vi "Load Temp.vi"(8 "error in (no error)":errorcluster, 10 "temp file name":string="ic_sparc.cfg", 11 "Channel in":refnum<class "Channel.lvclass">) -> (0 "error out":errorcluster, 3 "Channel out":refnum<class "Channel.lvclass">)   [LabVIEW 2018, in "Channel.lvclass"]
uses:
  Channel.lvclass
  Channel.lvclass/Channel.ctl
  <vilib>/Utility/config.llb/Read Key (String).vi
  Interface/Interface.lvclass
  <vilib>/Utility/config.llb/NI_LVConfig.lvlib
panel:
  in  "Temp cluster":T1={"COOLER_POWER_STATUS"=0, "CURRENT_TEMPERATURE"=20} {"CURRENT_TEMPERATURE" min=0 max=0; "COOLER_POWER_STATUS" items=["Cooler OFF", "Cooler ON"]}
  out "file created?":bool
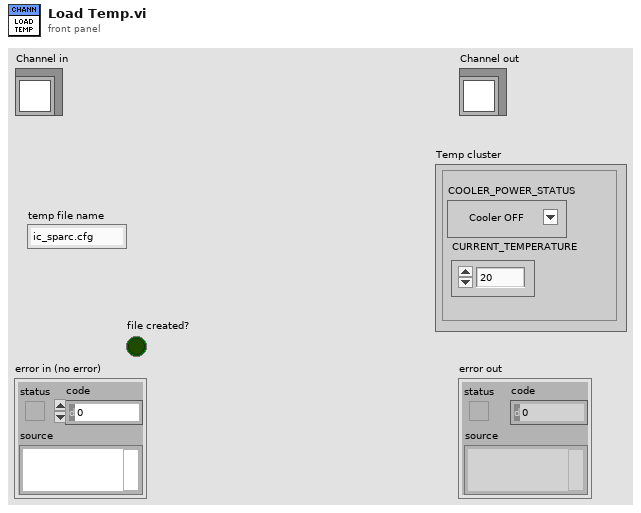
[diagram p1: front panel]
types:
  T1 = cluster{"COOLER_POWER_STATUS":i16, "CURRENT_TEMPERATURE":i8}
  T2 = typedef "NI_LVConfig.lvlib/Config Data RefNum.ctl" = refnum<k1>
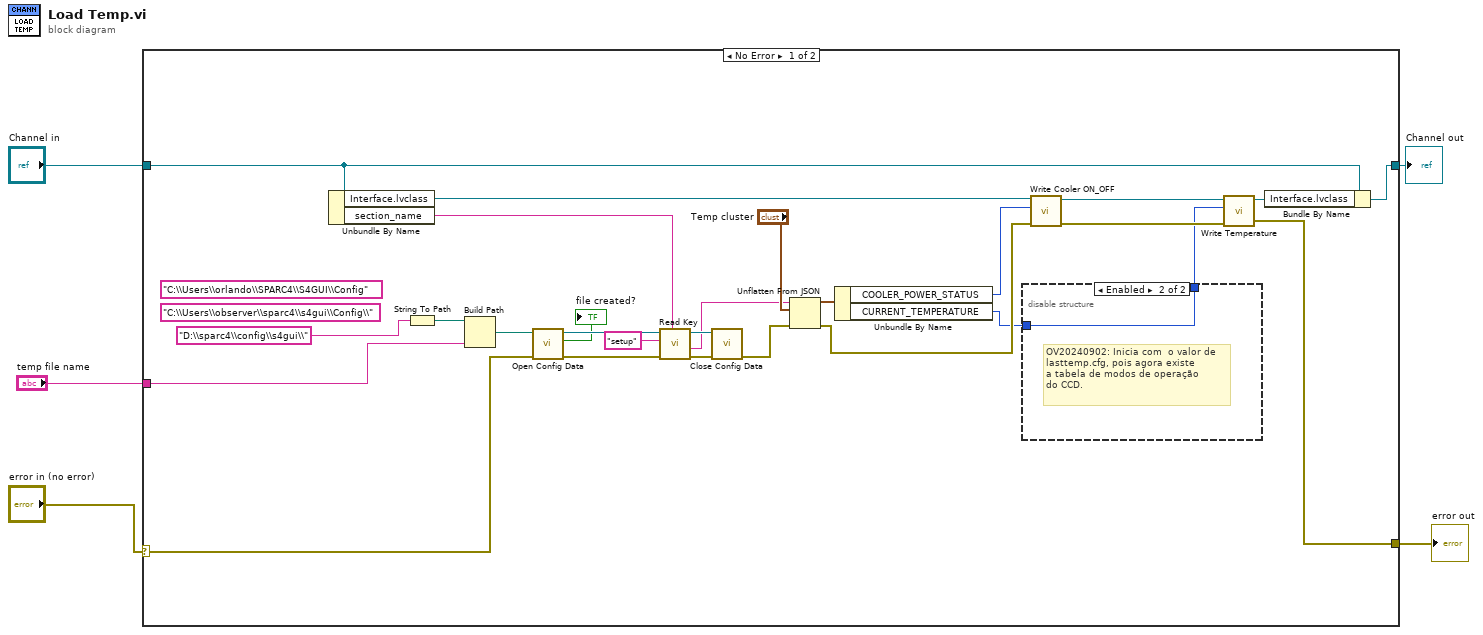
[diagram p0: block diagram]
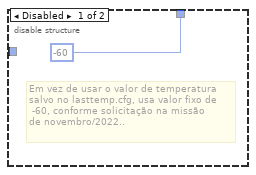
[diagram p2: hidden frame]
diagram:
  n1 = case shown="No Error" "error in (no error)" {
    selector: "error in (no error)" -> [w26 w36]
    tunnel: [w13 w36] -> w1
    tunnel: [w27 w35] -> w2
    tunnel: "Channel in" -> [w28 w35]
    tunnel: "temp file name" -> [w8 _]
    frame No Error {
      (unwired) "C:\\Users\\observer\\sparc4\\s4gui\\Config\\" ("string")
      (unwired) "C:\\Users\\orlando\\SPARC4\\S4GUI\\Config"
      n2 = Unbundle By Name(w28) -> ("Interface.lvclass"=w21:refnum<class "Interface.lvclass">, "section_name"=w31:string)
      n3 = String To Path(string="D:\\sparc4\\config\\s4gui\\") -> (path=w7:path)
      n4 = Build Path(base path=w7, name or relative path=w8) -> (appended path=w32:path)
      n5 = call <vilib>:"Open Config Data.vi"("error in (no error)"=w26, "configuration file path"=w32) -> ("error out"=w25:errorcluster, "file created?"=→"file created?":bool, "refnum"=w30:T2)  [unwired: 7 in]
      n6 = call-poly <vilib>:"Read Key.vi"("section"=w31, "error in (no error)"=w25, "key"="setup", "refnum"=w30) -> ("error out"=w22:errorcluster, "value"=w19:string, "refnum out"=w23:T2)  [unwired: 4 in, 1 out]
      n7 = call <vilib>:"Close Config Data.vi"("error in (no error)"=w22, "refnum"=w23) -> ("error out"=w12:errorcluster)  [unwired: 8 in, 1 out]
      n8 = Unflatten From JSON(JSON string=w19, type and defaults="Temp cluster", error in (no error)=w12) -> (value=w18:T1, error out=w11:errorcluster)  [unwired: 4 in]
      n9 = Unbundle By Name(w18) -> ("COOLER_POWER_STATUS"=w17:i16, "CURRENT_TEMPERATURE"=w9:i8)
      n10 = disable-structure shown="Enabled" {
        disable-tunnel: [i8 -60 w34] -> w10
        disable-tunnel: w9 -> [_ w34]
        frame Disabled {
          # "Em vez de usar o valor de temperatura \nsalvo no lasttemp.cfg, usa valor fixo de\n -60, conforme solicitação na missão \nde novembro/2022.."
        }
        frame Enabled {
          # "OV20240902: Inicia com  o valor de\nlasttemp.cfg, pois agora existe\na tabela de modos de operação\ndo CCD."
        }
      }
      n11 = call-dynamic "Write Cooler ON_OFF.vi"("error in (no error)"=w11, "Cooler ON/OFF"=w17, "Interface in"=w21) -> ("error out"=w14:errorcluster, "Interface out"=w16:refnum<class "Interface.lvclass">)  [unwired: 7 in]
      n12 = call-dynamic "Write Temperature.vi"("error in (no error)"=w14, "Temperature"=w10, "Interface in"=w16) -> ("error out"=w13:errorcluster, "Interface out"=w15:refnum<class "Interface.lvclass">)  [unwired: 7 in]
      n13 = Bundle By Name(cluster=w28, "Interface.lvclass"=w15) -> (w27:refnum<class "Channel.lvclass">)
    }
    frame Error {
    }
  }
  "error out" <- w1
  "Channel out" <- w2
